vi "shift_regsiter.vi"() -> ()   [LabVIEW 2017]
panel:
  out "Counter 2":i32[](array[numeric])
  out "counter":i32[](array[numeric])
  out "Array 2":dbl[](array[numeric])
  out "Array":dbl[](array[numeric])
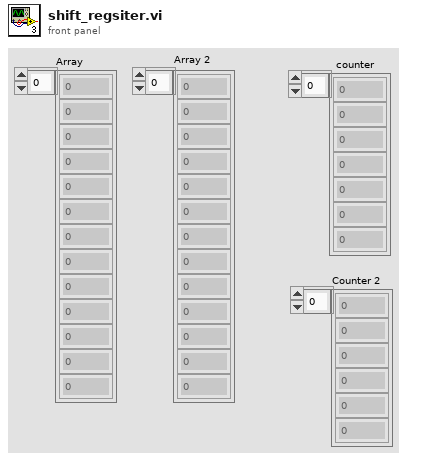
[diagram p1: front panel]
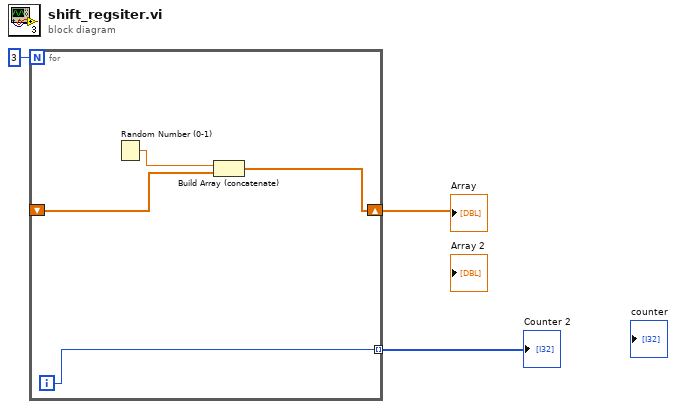
[diagram p0: block diagram]
diagram:
  n1 = for {
    N: 3 -> [_]
    shift-right: [w5] -> w2
    shift-left: _ -> [w7]
    tunnel: [w4] -> w1 mode=indexing
    i -> [w4]
    n2 = Random Number (0-1)() -> (number: 0 to 1=w6:dbl)
    n3 = Build Array (concatenate)(w6, w7) -> (w5:dbl[])
  }
  "Array" <- w2
  "Counter 2" <- w1
